vi "Drive Controller.vi"(8 "error in":errorcluster) -> ()   [LabVIEW 2019]
doc: "This VI executes continuously carrying out the current operation and responding to updates or new operation requests. It will often contain the timing or control code that is difficult to place directly in TeleOp. This VI generally opens all sensors and motors and isolates the rest of the robot code from knowing implementation details of how the operations are carried out."
uses:
  Drive Operations.ctl
  Drive Setpoints.ctl
  <vilib>/Rock Robotics/WPI/ThirdParty/REV Robotics/SPARK MAX/Typedef/Spark MAX Control Type.ctl
  <vilib>/Rock Robotics/WPI/Solenoid/WPI_SolenoidOpenDouble.vi
  <vilib>/Rock Robotics/WPI/Solenoid/WPI_SolenoidChannel.ctl
  <vilib>/Rock Robotics/WPI/Solenoid/WPI_SolenoidValue.ctl
  <vilib>/Rock Robotics/WPI/Solenoid/WPI_SolenoidSetEnum.vi
  2020 Robot/Framework/Robot Global Data.vi
  <vilib>/Rock Robotics/SystemInterfaces/AI/FPGA_AIChannel.ctl
  <vilib>/Rock Robotics/WPI/Ultrasonic/WPI_SonarMB1010AnalogOpen.vi
  <vilib>/Rock Robotics/WPI/Ultrasonic/WPI_SonarMB1010AnalogGetRange.vi
  <vilib>/ptbypt/NI_PtbyPt.lvlib
  Support Code/ADIS16448 IMU/ADIS16448_IMU.lvlib
  <vilib>/picture/picture.llb/imagedata.ctl
  Bordeaux/Command Stuff/Single Cmd Info.ctl
  <vilib>/Rock Robotics/WPI/Framework/Completion Status.ctl
panel:
  in  "PID gains M":T1={"proportional gain (Kc)"=0.02, "integral time (Ti, min)"=0.0, "derivative time (Td, min)"=0.0}
  out "Filtered x":dbl format="%0.2f"
  out "Current Angle":dbl
  out "Ball AA X":dbl
  in  "Interactive Values":T2
  in  "Buttons":cluster{"Execute Cmd":bool, "Abort Cmd":bool}
  out "Command Timing":cluster{"Start Time (ms)":u32, "Iterations":i32}
  out "Status":T6
  out "Current\nCmd":string
  # "Tip: The graph shows the motor setpoints. It may also be helpful to observe inputs and sensor values.\nYou may also want to display tuning or debugging controls."
  # "Interactive Command: You may fill in the settings for a command\nand schedule it with the Execute button. You can observe and abort\nany command while fine tuning the code for the controller."
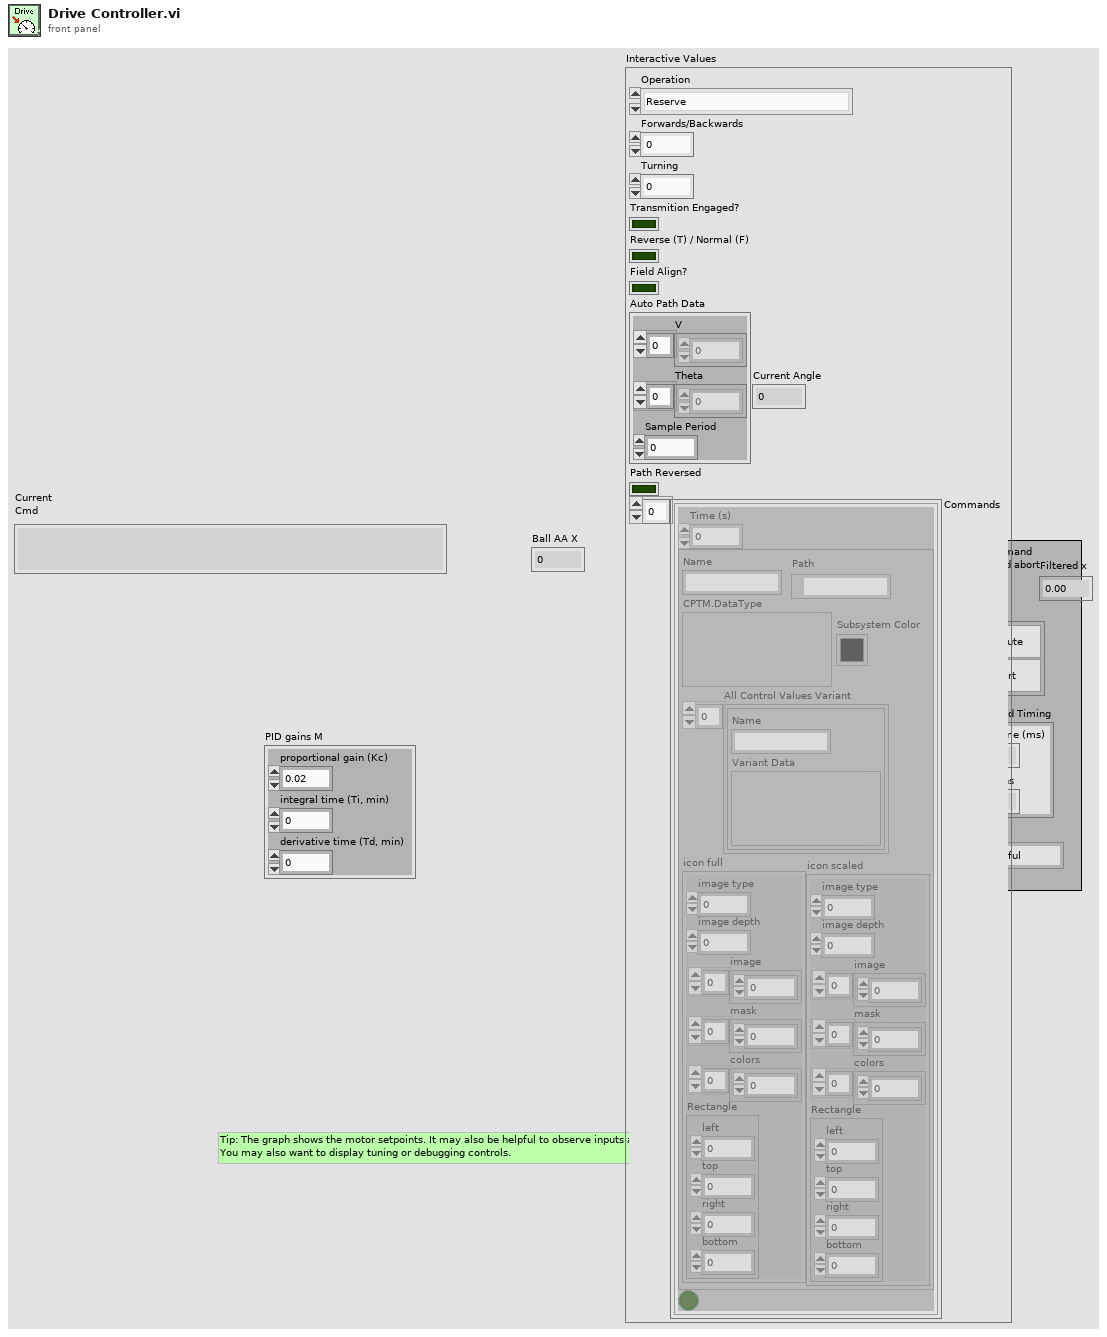
[diagram p1: front panel]
types:
  T1 = cluster{"proportional gain (Kc)":dbl, "integral time (Ti, min)":dbl, "derivative time (Td, min)":dbl}
  T2 = typedef "Drive Setpoints.ctl" = cluster{"Operation":T3, "Forwards/Backwards":dbl, "Turning":dbl, "Transmition Engaged?":bool, "Reverse (T) / Normal (F)":bool, "Field Align?":bool, "Auto Path Data":cluster{"V":dbl[], "Theta":dbl[], "Sample Period":dbl}, "Path Reversed":bool, "Commands":cluster{"Time (s)":dbl, T4, bool}[]}
  T3 = typedef "Drive Operations.ctl" = enum16{"Reserve", "Read Current", "Immediate", "Pod Racer", "Ball AA", "Play Back From Log"}
  T4 = typedef "Single Cmd Info.ctl" = cluster{"Name":string, "CPTM.DataType":variant, "All Control Values Variant":cluster{"Name":string, "Variant Data":variant}[], "icon full":T5, "icon scaled":T5, "Path":path, "Subsystem Color":u32}
  T5 = typedef "imagedata.ctl" = cluster{"image type":i32, "image depth":i32, "image":u8[], "mask":u8[], "colors":u32[], "Rectangle":cluster{"left":i16, "top":i16, "right":i16, "bottom":i16}}
  T6 = typedef "Completion Status.ctl" = enum16{"Successful", "Aborted", "Incomplete"}
  T7 = cluster{"P Gain":dbl, "I Gain":dbl, "D Gain":dbl, "F Gain":dbl, "I Zone":dbl, "Min Output":dbl, "Max Output":dbl}
  T8 = typedef "FPGA_AIChannel.ctl" = enum8{"AI 0", "AI 1", "AI 2", "AI 3", "AI MXP 0", "AI MXP 1", "AI MXP 2", "AI MXP 3", "Invalid"}
  T9 = typedef "WPI_SolenoidChannel.ctl" = enum8{"Solenoid 0", "Solenoid 1", "Solenoid 2", "Solenoid 3", "Solenoid 4", "Solenoid 5", "Solenoid 6", "Solenoid 7", "Invalid"}
  T10 = typedef "ADIS16448_IMU.lvlib/ADI_IMU_ADIS16448_IMUDevRef.ctl" = cluster{"DevStatus":errorcluster, "Handle":i32, "SPI Bus":T11, "Device Found":bool, "Device Ready":bool, "Yaw Axis":enum16{"X", "Y", "Z"}, "AHRS Algorithm":enum16{"Complementary", "Madgwick"}, "Serial":u16, "Lot ID 2":u16, "Lot ID 1":u16, "Bytes Per Sample":u16, "Calibrate On Open?":bool}
  T11 = typedef "spi_bus.ctl" = enum16{"SPI On-Board, CS0", "SPI On-Board, CS1", "SPI On-Board, CS2", "SPI On-Board, CS3", "SPI MXP", "Invalid"}
  T12 = typedef "WPI_SonarMB1010AnalogDeviceRef.ctl" = cluster{"AIDeviceRef":T13, "Scaling factor (V/in)":dbl, "Average Bits":u8}
  T13 = typedef "WPI_AnalogChannelDevRef.ctl" = cluster{"DevStatus":errorcluster, "Analog Channel":T8}
  T14 = typedef "WPI_SolenoidDevRef.ctl" = cluster{"DevStatus":errorcluster, "Pneumatics Control Module":u8, "Forward Solenoid Channel":T9, "Reverse Solenoid Channel":T9}
  T15 = typedef "Command Status Info.ctl" = cluster{"Name":string, "Status":T6, "notifier out":T16}
  T16 = typedef "Completion Notifier.ctl" = refnum<notifier>
  T17 = cluster{"SubSystem Data":T2, cluster{"Start Time (ms)":u32, "Iterations":i32}, cluster{"Command Info":T15, "Description":string, "Default Command":T2, "queue out":refnum<queue>, "Subsystem Name":string}}
  T18 = typedef "Spark MAX Control Type.ctl" = enum16{"Percent VBus", "Voltage", "Velocity", "Position", "Smart Motion", "Current", "Smart Velocity"}
  T19 = typedef "WPI_SolenoidValue.ctl" = enum16{"Off", "On", "Forward", "Reverse"}
  T20 = enum16{"MAX 90", "Pod Racer", "MAX 180", "Turn to Home", "Turn to Rocket", "Auto-Align", "Turn to ..."}
  T21 = cluster{"V":dbl[], "Theta":dbl[], "Sample Period":dbl}
  T22 = cluster{"X Angle":dbl, "Y Angle":dbl, "Z Angle":dbl}
  T23 = cluster{"SubSystem Data":T2, cluster{"Start Time (ms)":u32, "Iterations":i32}, "Default Command Arguments":cluster{"Command Info":T15, "Description":string, "Default Command":T2, "queue out":refnum<queue>, "Subsystem Name":string}}
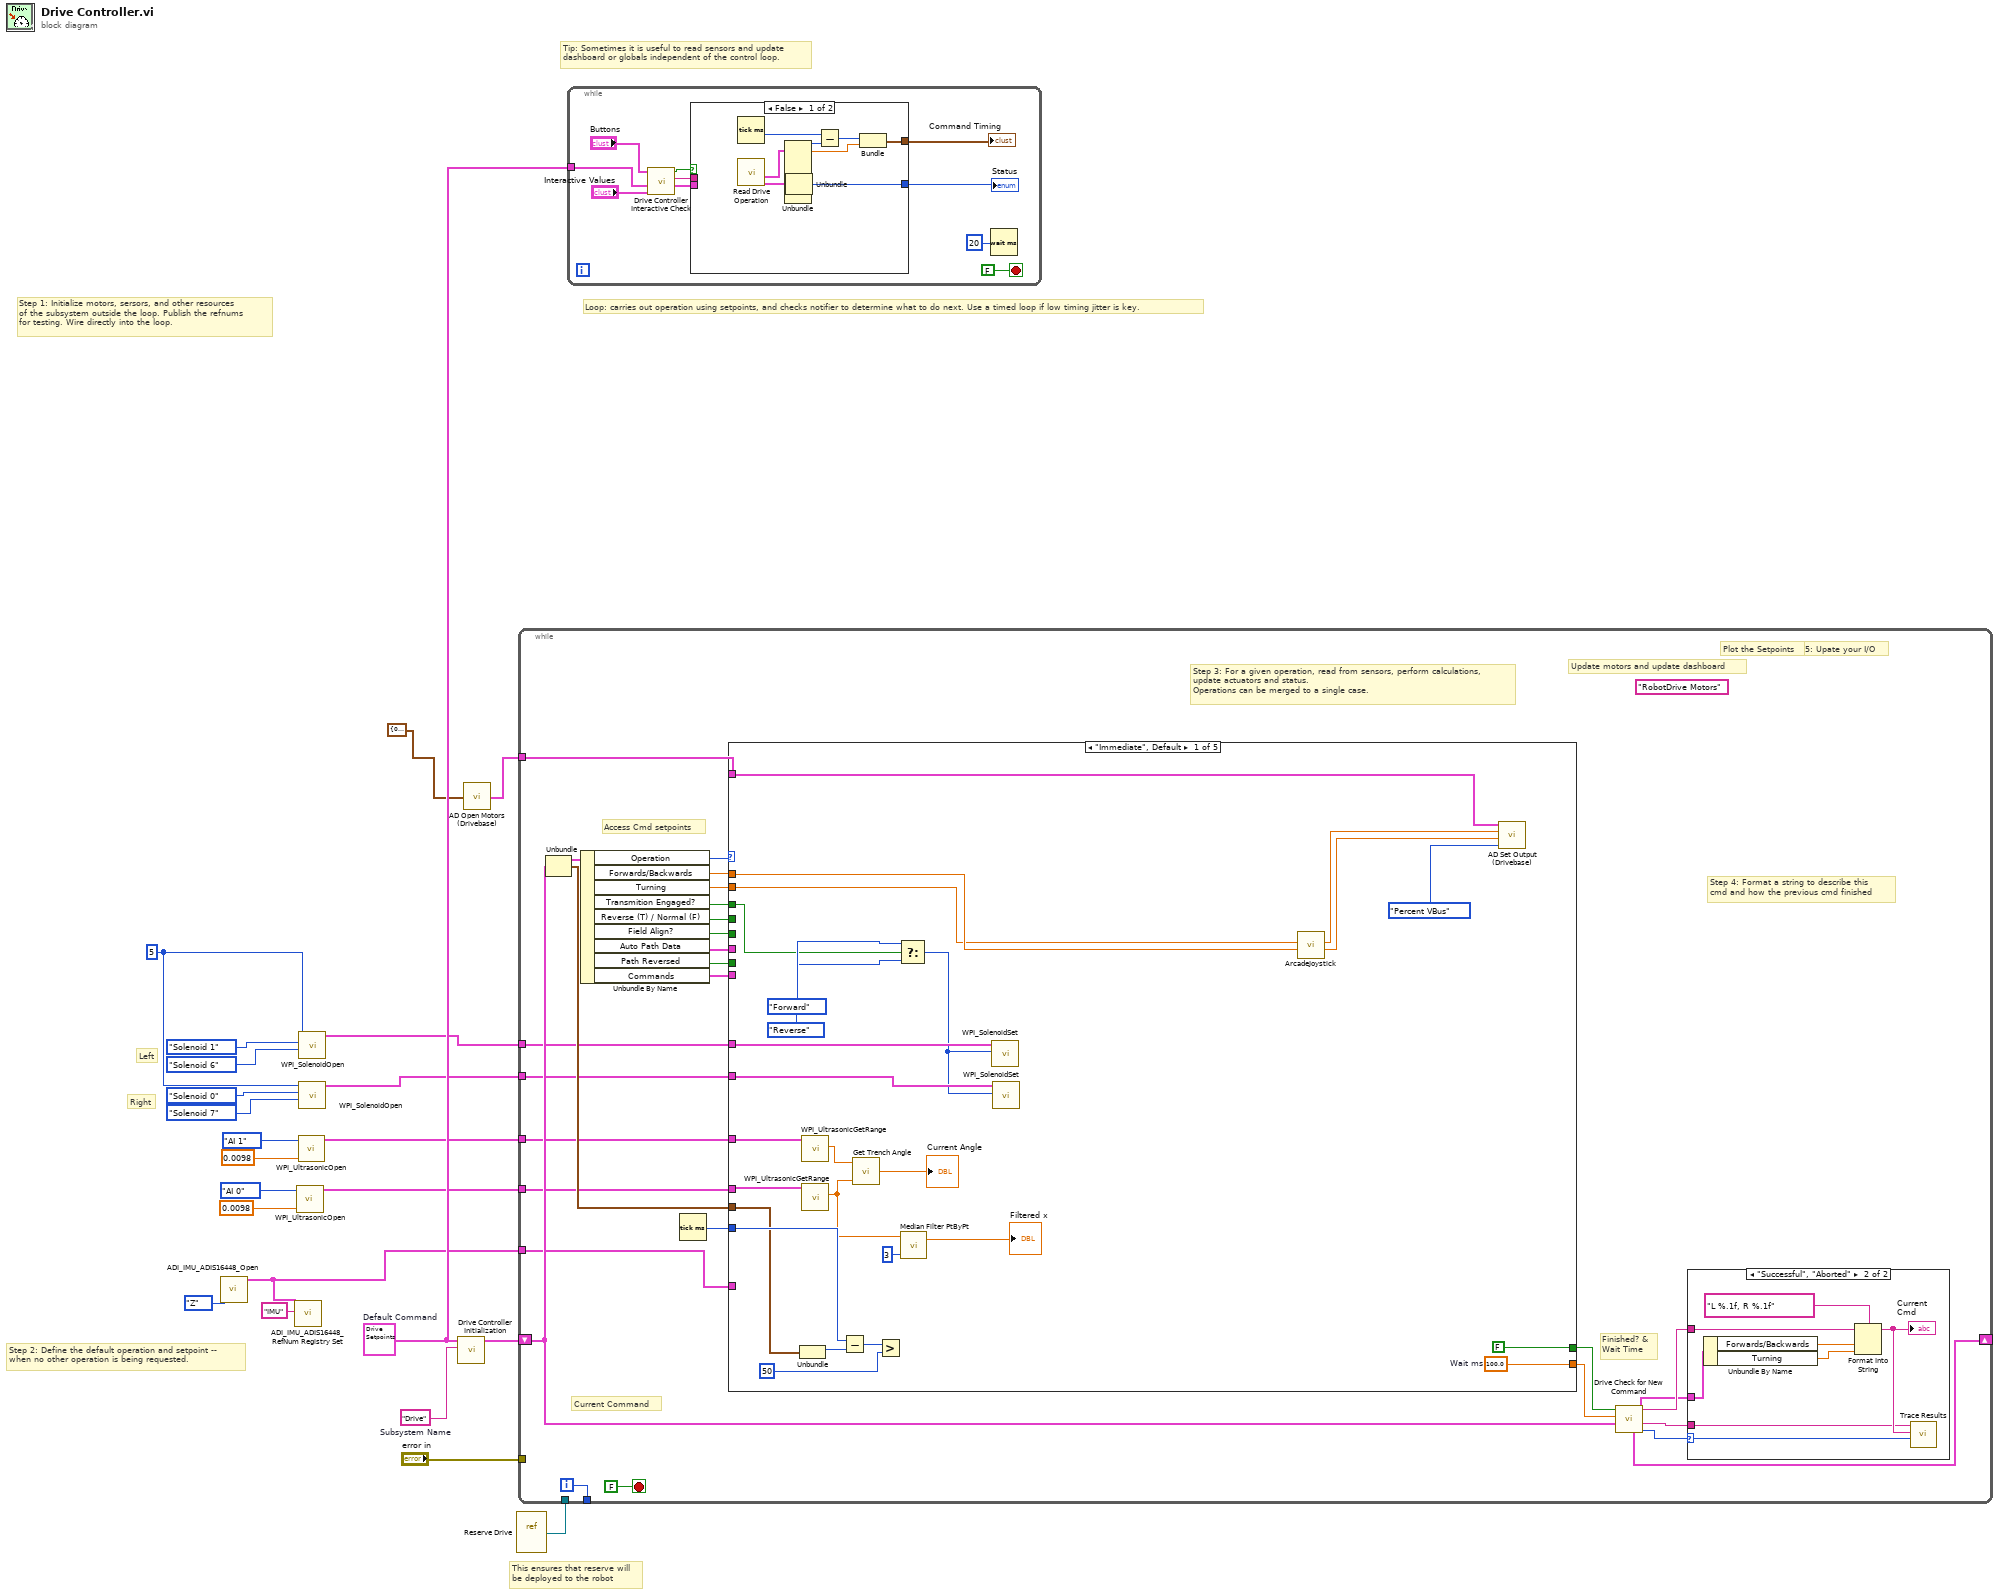
[diagram p0: block diagram]
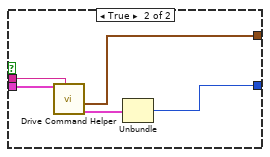
[diagram p2: hidden frame]
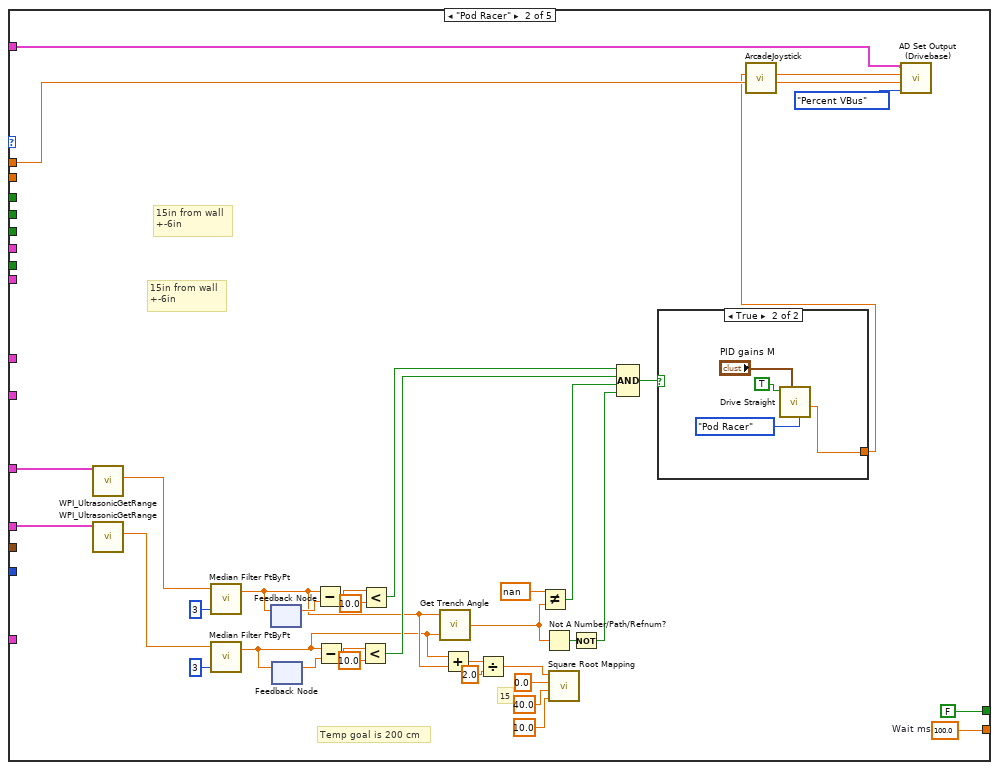
[diagram p4: hidden frame]
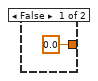
[diagram p5: hidden frame]
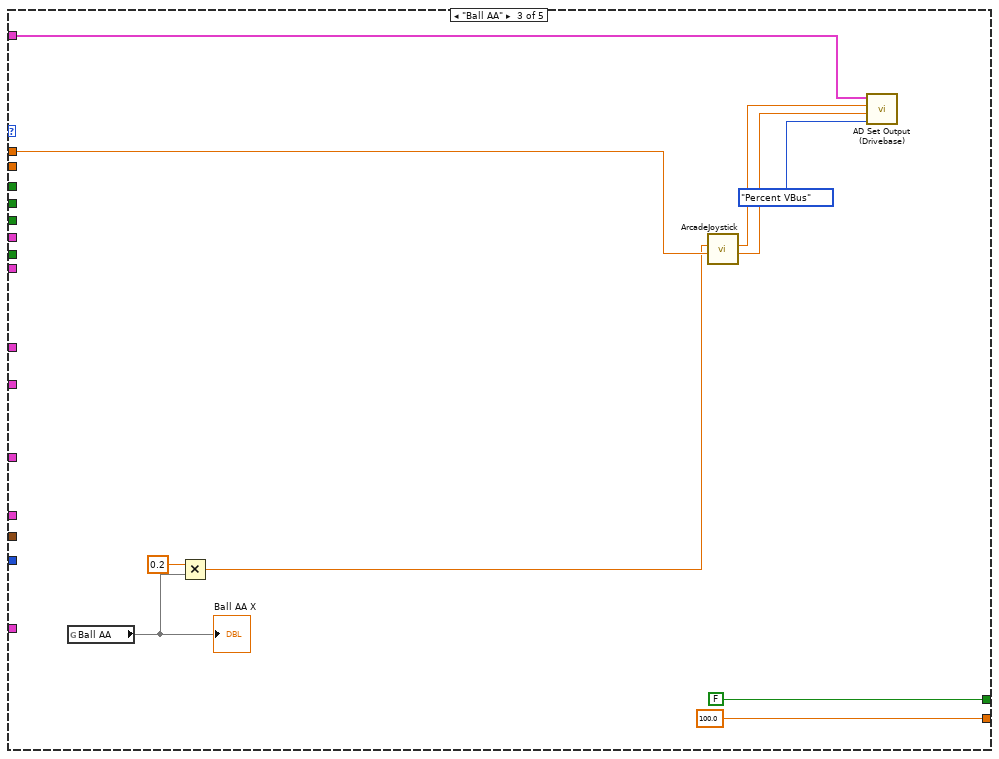
[diagram p6: hidden frame]
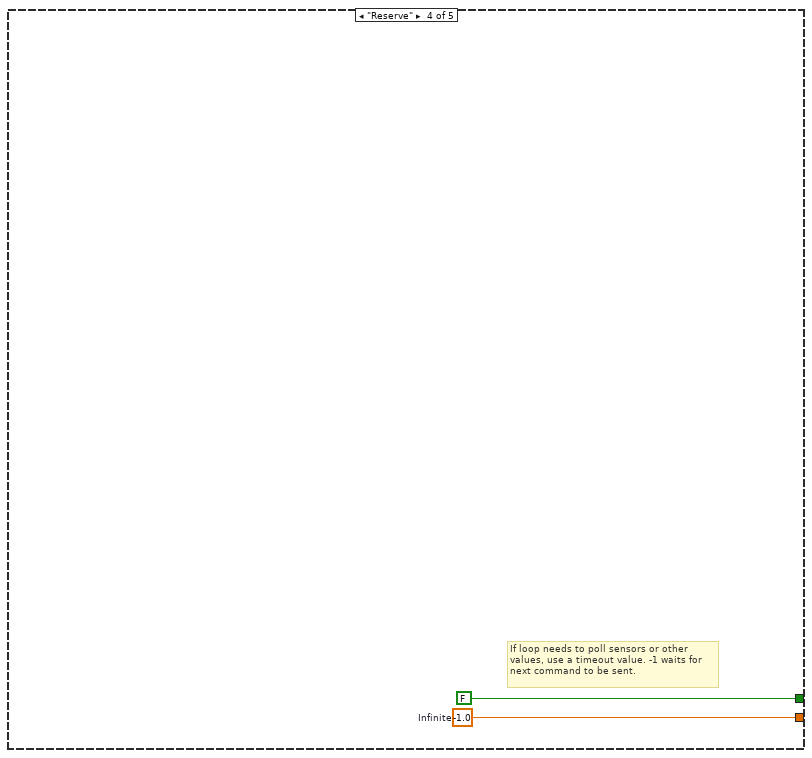
[diagram p7: hidden frame]
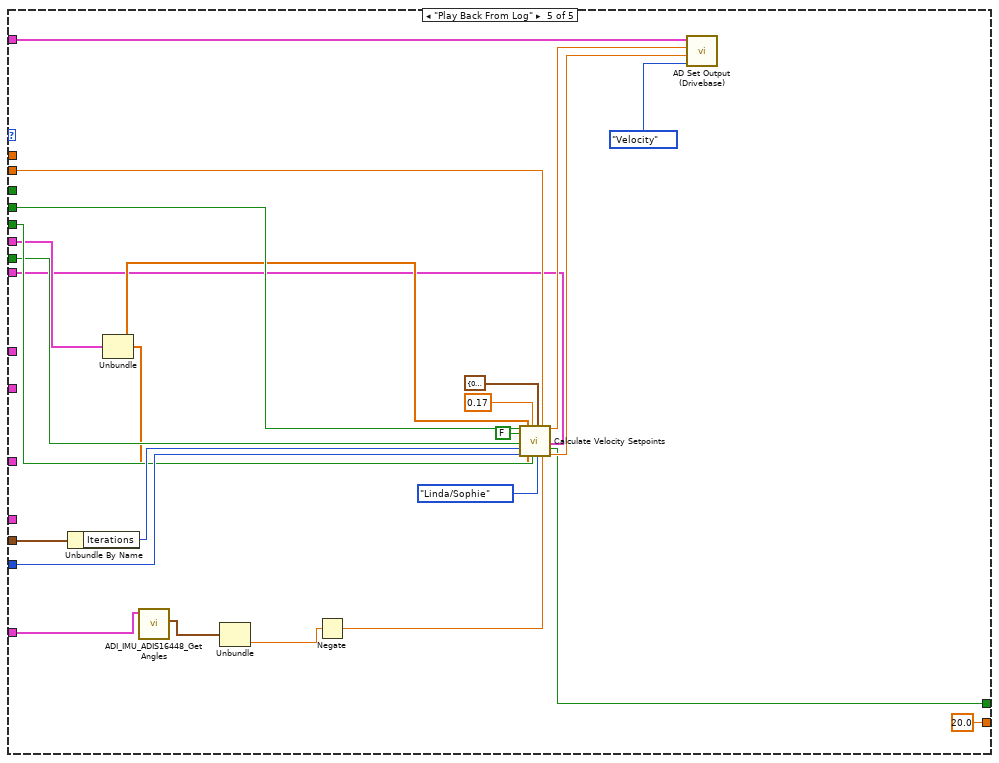
[diagram p8: hidden frame]
diagram:
  w18 = u8 5 ("Pneumatics Control Module (0)")
  w19 = T2 {"Operation"=enum."Immediate", "Forwards/Backwards"=0.0, "Turning"=0.0, "Transmition Engaged?"=FALSE, "Reverse (T) / Normal (F)"=FALSE, "Field Align?"=FALSE, "Auto Path Data"={"V"=[], "Theta"=[], "Sample Period"=0.0}, "Path Reversed"=FALSE, "Commands"=[]}  # Default Command
  w23 = "Drive"  # Subsystem Name
  # "Left"
  # "Right"
  # "This ensures that reserve will\nbe deployed to the robot"
  # "Tip: Sometimes it is useful to read sensors and update\ndashboard or globals independent of the control loop."
  # "Step 2: Define the default operation and setpoint --\nwhen no other operation is being requested."
  # "Step 1: Initialize motors, sersors, and other resources\nof the subsystem outside the loop. Publish the refnums\nfor testing. Wire directly into the loop."
  # "Loop: carries out operation using setpoints, and checks notifier to determine what to do next. Use a timed loop if low timing jitter is key."
  n1 = call "ADI_IMU_ADIS16448_Open.vi"("Yaw Axis"=enum16{"X", "Y", "Z"}."Z") -> ("ADI IMU DevRef Out"=w2:T10)  [unwired: 9 in, 1 out]
  n2 = call "ADI_IMU_ADIS16448_RefNum Registry Set.vi"("refnum name"="IMU", "ADI IMU DevRef"=w2) -> ()  [unwired: 8 in, 2 out]
  n3 = call-poly <vilib>:"WPI_UltrasonicOpen.vi"("Scaling factor (V/in)"=0.0098, "Analog Channel"=FPGA_AIChannel."AI 0") -> ("SonarMB1010AnalogDevRef"=w6:T12)  [unwired: 8 in, 1 out]
  n4 = call-poly <vilib>:"WPI_UltrasonicOpen.vi"("Scaling factor (V/in)"=0.0098, "Analog Channel"=FPGA_AIChannel."AI 1") -> ("SonarMB1010AnalogDevRef"=w11:T12)  [unwired: 8 in, 1 out]
  n5 = call-poly <vilib>:"WPI_SolenoidOpen.vi"("Reverse Solenoid Channel"=WPI_SolenoidChannel."Solenoid 6" ("Forward Solenoid Channel"), "Forward Solenoid Channel"=WPI_SolenoidChannel."Solenoid 1", "Pneumatics Control Module (0)"=w18) -> ("SolenoidDevRef"=w13:T14)  [unwired: 7 in, 1 out]
  n6 = call-poly <vilib>:"WPI_SolenoidOpen.vi"("Reverse Solenoid Channel"=WPI_SolenoidChannel."Solenoid 7" ("Forward Solenoid Channel"), "Forward Solenoid Channel"=WPI_SolenoidChannel."Solenoid 0", "Pneumatics Control Module (0)"=w18) -> ("SolenoidDevRef"=w12:T14)  [unwired: 7 in, 1 out]
  n7 = call "Drive Controller Initialization.vi"("Subsystem Name"=w23, "Default Command"=w19) -> ("Current Command"=w21:T17)  [unwired: 9 in]
  n8 = call "AD Open Motors (Drivebase).vi"("PID Constants for Sparks"=T7 {"P Gain"=0.00035, "I Gain"=5e-07, "D Gain"=0.0, "F Gain"=0.0002, "I Zone"=0.0, "Min Output"=-1.0, "Max Output"=1.0}) -> ("output cluster"=w5:cluster{"Left":string[], "Right":string[]})
  n9 = vi-ref "Reserve Drive.vi"() -> (w20:refnum<vi>)
  n10 = while {
    shift-right: [w43] -> _
    shift-left: w21 -> [w36]
    tunnel: [w50] -> _
    tunnel: "error in" -> [_]
    tunnel: w20 -> [_]
    tunnel: w13 -> [w34]
    tunnel: w12 -> [w33]
    tunnel: w11 -> [w32]
    tunnel: w6 -> [w31]
    tunnel: w5 -> [w30]
    tunnel: w2 -> [w24]
    i -> [w50]
    stop <- FALSE stop-if-true
    (unwired) "RobotDrive Motors" ("Name")
    # "Step 5: Upate your I/O"
    # "Step 4: Format a string to describe this\ncmd and how the previous cmd finished"
    # "Current Command"
    # "Update motors and update dashboard"
    # "Plot the Setpoints"
    # "Access Cmd setpoints"
    # "Finished? &\nWait Time"
    # "Step 3: For a given operation, read from sensors, perform calculations,\nupdate actuators and status.\nOperations can be merged to a single case."
    n11 = Unbundle(w36) -> ("SubSystem Data"=w49:T2, w37:cluster{"Start Time (ms)":u32, "Iterations":i32})  [unwired: 1 out]
    n12 = Unbundle By Name(w49) -> ("Operation"=w48:T3, "Forwards/Backwards"=w47:dbl, "Turning"=w46:dbl, "Transmition Engaged?"=w35:bool, "Reverse (T) / Normal (F)"=w29:bool, "Field Align?"=w28:bool, "Auto Path Data"=w26:T21, "Path Reversed"=w27:bool, "Commands"=w25:cluster{"Time (s)":dbl, T4, bool}[])
    n13 = Tick Count (ms)() -> (millisecond timer value=w45:u32)
    n14 = case shown="\"Immediate\", Default" w48 {
      tunnel: [w85 w120 100.0 ("Infinite") w138 20.0 ("Infinite")] -> w42
      tunnel: [FALSE ("ignore previous (F)") FALSE ("ignore previous (F)") FALSE ("ignore previous (F)") FALSE ("ignore previous (F)") w149] -> w41
      tunnel: w37 -> [w80 _ _ _ w157]
      tunnel: w47 -> [w72 w115 w136 _ _]
      tunnel: w46 -> [w71 _ _ _ w150]
      tunnel: w45 -> [w81 _ _ _ w155]
      tunnel: w35 -> [w74 _ _ _ _]
      tunnel: w34 -> [w78 _ _ _ _]
      tunnel: w33 -> [w77 _ _ _ _]
      tunnel: w32 -> [w69 w89 _ _ _]
      tunnel: w31 -> [w68 w88 _ _ _]
      tunnel: w30 -> [w63 w119 w133 _ w162]
      tunnel: w29 -> [_ _ _ _ w152]
      tunnel: w28 -> [_ _ _ _ w154]
      tunnel: w27 -> [_ _ _ _ w153]
      tunnel: w26 -> [_ _ _ _ w148]
      tunnel: w24 -> [_ _ _ _ w144]
      tunnel: w25 -> [_ _ _ _ w139]
      frame "Immediate", Default {
        w85 = 100.0  # Wait ms
        n15 = Unbundle(w80) -> ("Start Time (ms)"=w82:u32)  [unwired: 1 out]
        n16 = call-poly <vilib>:"WPI_UltrasonicGetRange.vi"("SonarMB1010AnalogDevRef"=w69) -> ("Distance"=w70:dbl)  [unwired: 8 in, 2 out]
        n17 = call-poly <vilib>:"WPI_UltrasonicGetRange.vi"("SonarMB1010AnalogDevRef"=w68) -> ("Distance"=w65:dbl)  [unwired: 8 in, 2 out]
        n18 = Subtract(x=w81, y=w82) -> (x-y=w83:u32)
        n19 = call "Get Trench Angle.vi"("Distance 2"=w65, "Distance 1"=w70) -> ("Current Angle"=→"Current Angle":dbl)  [unwired: 1 in]
        n20 = Greater?(x=w83, y=u8 50 ("Left Motor")) -> ()  [unwired: 1 out]
        n21 = Select(t=WPI_SolenoidValue."Forward" ("Value"), s=w74, f=WPI_SolenoidValue."Reverse" ("Value")) -> (s? t:f=w73:T19)
        n22 = call <vilib>:"Median Filter PtByPt.vi"("rank"=3, "x"=w65) -> ("Filtered x"=→"Filtered x":dbl)  [unwired: 2 in, 1 out]
        n23 = call-poly <vilib>:"WPI_SolenoidSet.vi"("Value"=w73, "SolenoidDevRef"=w78) -> ()  [unwired: 8 in, 2 out]
        n24 = call-poly <vilib>:"WPI_SolenoidSet.vi"("Value"=w73, "SolenoidDevRef"=w77) -> ()  [unwired: 8 in, 2 out]
        n25 = call "ArcadeJoystick.vi"("Y axis value"=w72, "X axis value"=w71) -> ("Right Motor Value"=w61:dbl, "Left Motor Value"=w62:dbl)  [unwired: 8 in]
        n26 = call "AD Set Output (Drivebase).vi"("Control Mode"=Spark_MAX_Control_Type."Percent VBus", "Right"=w61, "Left"=w62, "Input cluster"=w63) -> ()
      }
      frame "Pod Racer" {
        w120 = 100.0  # Wait ms
        # "15"
        # "15in from wall\n+-6in"
        # "Temp goal is 200 cm"
        # "15in from wall\n+-6in"
        n27 = call-poly <vilib>:"WPI_UltrasonicGetRange.vi"("SonarMB1010AnalogDevRef"=w89) -> ("Distance"=w94:dbl)  [unwired: 8 in, 2 out]
        n28 = call-poly <vilib>:"WPI_UltrasonicGetRange.vi"("SonarMB1010AnalogDevRef"=w88) -> ("Distance"=w91:dbl)  [unwired: 8 in, 2 out]
        n29 = call <vilib>:"Median Filter PtByPt.vi"("rank"=3, "x"=w94) -> ("Filtered x"=w95:dbl)  [unwired: 2 in, 1 out]
        n30 = call <vilib>:"Median Filter PtByPt.vi"("rank"=3, "x"=w91) -> ("Filtered x"=w92:dbl)  [unwired: 2 in, 1 out]
        n31 = feedback #1() -> (w111:dbl)  [unwired: 1 in]
        n32 = feedback-in #1(w95) -> ()
        n33 = feedback #2() -> (w110:dbl)  [unwired: 1 in]
        n34 = feedback-in #2(w92) -> ()
        n35 = Subtract(x=w95, y=w111) -> (x-y=w107:dbl)
        n36 = Subtract(x=w92, y=w110) -> (x-y=w104:dbl)
        n37 = Less?(x=w104, y=10.0) -> (x < y?=w105:bool)
        n38 = Less?(x=w107, y=10.0) -> (x < y?=w109:bool)
        n39 = call "Get Trench Angle.vi"("Distance 2"=w92, "Distance 1"=w95) -> ("Current Angle"=w90:dbl)  [unwired: 1 in]
        n40 = Add(x=w92, y=w95) -> (x+y=w114:dbl)
        n41 = Divide(x=w114, y=2.0) -> (x/y=w103:dbl)
        n42 = Not Equal?(x=nan, y=w90) -> (x != y?=w112:bool)
        n43 = Not A Number/Path/Refnum?(number/path/refnum=w90) -> (NaN/Path/Refnum?=w100:bool)
        n44 = call "Square Root Mapping.vi"("x"=w103, "Min Distance"=0.0 ("Min A"), "Max Distance"=40.0 ("Max A"), "Angle"=10.0 ("Max B")) -> ()  [unwired: 4 in, 1 out]
        n45 = Not(x=w100) -> (.not. x?=w99:bool)
        n46 = Compound Arithmetic op=AND(w109, w105, w112, w99) -> (w87:bool)
        n47 = case shown="True" w87 {
          tunnel: [0.0 ("Turn Setpoint") w126] -> w86
          frame False {
          }
          frame True {
            n48 = call "Drive Straight.vi"("Maneuver"=T20."Pod Racer", "PID gains M"="PID gains M", "Enable?"=TRUE) -> ("Turn Setpoint"=w126:dbl)  [unwired: 8 in]
          }
        }
        n49 = call "ArcadeJoystick.vi"("Y axis value"=w115, "X axis value"=w86) -> ("Right Motor Value"=w117:dbl, "Left Motor Value"=w118:dbl)  [unwired: 8 in]
        n50 = call "AD Set Output (Drivebase).vi"("Control Mode"=Spark_MAX_Control_Type."Percent VBus", "Right"=w117, "Left"=w118, "Input cluster"=w119) -> ()
      }
      frame "Ball AA" {
        n51 = global read "Robot Global Data.vi" "Ball AA"() -> (w129)
        "Ball AA X" <- w129
        n52 = Multiply(x=0.2, y=w129) -> (x*y=w127:dbl)
        n53 = call "ArcadeJoystick.vi"("Y axis value"=w136, "X axis value"=w127) -> ("Right Motor Value"=w130:dbl, "Left Motor Value"=w132:dbl)  [unwired: 8 in]
        n54 = call "AD Set Output (Drivebase).vi"("Control Mode"=Spark_MAX_Control_Type."Percent VBus", "Right"=w130, "Left"=w132, "Input cluster"=w133) -> ()
      }
      frame "Reserve" {
        w138 = -1.0  # Infinite
        # "If loop needs to poll sensors or other\nvalues, use a timeout value. -1 waits for\nnext command to be sent."
      }
      frame "Play Back From Log" {
        n55 = Unbundle By Name(w157) -> ("Iterations"=w156:i32)
        n56 = Unbundle(w148) -> ("V"=w147:dbl[], "Theta"=w146:dbl[])  [unwired: 1 out]
        n57 = call "ADI_IMU_ADIS16448_Get Angles.vi"("ADI IMU DevRef"=w144) -> ("IMU Angles Out"=w143:T22)  [unwired: 7 in, 3 out]
        n58 = Unbundle(w143) -> ("Z Angle"=w142:dbl)  [unwired: 2 out]
        n59 = Negate(x=w142) -> (-x=w141:dbl)
        n60 = call "Calculate Velocity Setpoints.vi"("Negated"=w152, "Front is Back"=FALSE, "Reversed"=w153, "Iterations"=w156, "Time"=w155, "Velocity Data"=w147, "Angular Data (Relative)"=w146, "f"=0.17, "Align?"=w154, "PID gains L/S 2"=T1 {"proportional gain (Kc)"=0.08, "integral time (Ti, min)"=0.0, "derivative time (Td, min)"=0.001}, "Enum"=enum16{"Vantage", "Mule", "Linda/Sophie"}."Linda/Sophie", "Angle To Get"=w150, "IMU Input"=w141, "Commands"=w139) -> ("Left Setpoint"=w163:dbl, "Finished?"=w149:bool, "Right Setpoint"=w161:dbl)  [unwired: 1 in, 2 out]
        n61 = call "AD Set Output (Drivebase).vi"("Control Mode"=Spark_MAX_Control_Type."Velocity", "Right"=w161, "Left"=w163, "Input cluster"=w162) -> ()
      }
    }
    n62 = call "Drive Check for New Command.vi"("input cluster"=w36, "Wait time (ms)"=w42, "Finished?"=w41) -> ("Completion"=w44:T6, "Subsystem Name"=w38:string, "Current Command"=w39:T2, "Initial Trace String"=w40:string, "Next Command"=w43:T23)  [unwired: 4 in]
    n63 = case shown="\"Successful\", \"Aborted\"" w44 {
      selector: w44 -> [_ w59]
      tunnel: w40 -> [_ w54]
      tunnel: w39 -> [_ w55]
      tunnel: w38 -> [_ w52]
      frame "Incomplete", Default {
        # "Continuing current command"
      }
      frame "Successful", "Aborted" {
        # "Report and setup for next command"
        n64 = Unbundle By Name(w55) -> ("Forwards/Backwards"=w57:dbl, "Turning"=w58:dbl)
        n65 = Format Into String(format string="L %.1f, R %.1f", initial string=w54, w57, w58) -> (resulting string=w53:string)  [unwired: 1 in, 1 out]
        "Current\nCmd" <- w53
        n66 = call <vilib>:"Trace Results.vi"("Status of previous command"=w59, "Description"=w53, "Subsystem"=w52) -> ()  [unwired: 9 in]
      }
    }
  }
  n67 = while {
    tunnel: w19 -> [w165]
    stop <- FALSE stop-if-true
    n68 = call "Drive Controller Interactive Check.vi"("Interactive Command In"="Interactive Values", "Default Command"=w165, "Buttons"="Buttons") -> ("Interactive Command Out"=w167:T2, "Trace String"=w168:string, "Schedule"=w169:bool)  [unwired: 6 in]
    n69 = case shown="False" w169 {
      tunnel: [w178 w186] -> w170
      tunnel: [w177 w182] -> w171
      tunnel: w168 -> [_ w184]
      tunnel: w167 -> [_ w183]
      frame False {
        n70 = Tick Count (ms)() -> (millisecond timer value=w181:u32)
        n71 = call "Read Drive Operation.vi"() -> ("Command Info"=w175:T15, "SubSystem Data"=w174:T2)  [unwired: 9 in, 1 out]
        n72 = Unbundle(w174) -> ("Operation"=w179:T3, "Forwards/Backwards"=w176:dbl)  [unwired: 7 out]
        n73 = Unbundle(w175) -> ("Status"=w178:T6)  [unwired: 2 out]
        n74 = Subtract(x=w181, y=w179) -> (x-y=w180:u32)
        n75 = Bundle(w180, "Forwards/Backwards"=w176) -> (w177:cluster{u32, "Forwards/Backwards":dbl})  [unwired: 1 in]
      }
      frame True {
        n76 = call "Drive Command Helper.vi"("Description"=w184, "SubSystem Data"=w183) -> ("Command Info Out"=w185:T15, "Command Timing"=w182:cluster{"Start Time (ms)":u32, "Iterations":i32})  [unwired: 7 in, 1 out]
        n77 = Unbundle(w185) -> ("Status"=w186:T6)  [unwired: 2 out]
      }
    }
    "Status" <- w170
    "Command Timing" <- w171
    n78 = Wait (ms)(milliseconds to wait=u32 20) -> ()  [unwired: 1 out]
  }
